vi "Close.vi"(8 "error in (no error)":errorcluster, 11 "Channel in":refnum<class "Channel.lvclass">) -> (0 "error out":errorcluster)   [LabVIEW 2020, in "Nominal Streaming.lvlib" / "Channel.lvclass"]
uses:
  Channel.lvclass
  Channel.lvclass/Channel.ctl
  Stream/Stream.lvclass/Stream.ctl
  Stream/library.get.vi
  Stream/Stream.lvclass
  bin/lib_nominal-streaming-lv_64.dll
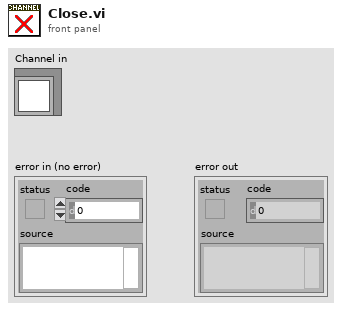
[diagram p1: front panel]
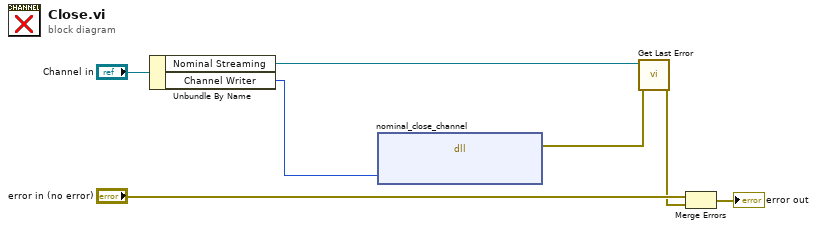
[diagram p0: block diagram]
diagram:
  n1 = Unbundle By Name("Channel in") -> ("Nominal Streaming"=w1:refnum<class "Stream.lvclass">, "Channel Writer"=w6:u64)
  n2 = dll-call lib="C:/code/nominal-streaming-labview-ffi/lv_src/bin/lib_nominal-streaming-lv_*.*" fn="nominal_close_channel"("writer_handle"=w6) -> (error out=w5:errorcluster)  [unwired: 5 in, 1 out]
  n3 = call "Get Last Error.vi"("error in (no error)"=w5, "Nominal Streaming in"=w1) -> ("error out"=w3:errorcluster)  [unwired: 8 in, 1 out]
  n4 = Merge Errors("error in (no error)", w3) -> (→"error out":errorcluster)
